vi "ControlShooter.vi"(1 "State":T2) -> (0 "To Shooter\nSolenoid Loop":T1=enum."Forward")   [LabVIEW 2013]
uses:
  typedefs/subStates.ctl
  <vilib>/Rock Robotics/WPI/Solenoid/WPI_SolenoidGetEnum.vi
  <vilib>/Rock Robotics/WPI/Solenoid/WPI_SolenoidValue.ctl
  typedefs/fg_typedef.ctl
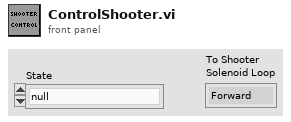
[diagram p1: front panel]
types:
  T1 = typedef "WPI_SolenoidValue.ctl" = enum16{"Off", "On", "Forward", "Reverse"}
  T2 = typedef "subStates.ctl" = enum16{"null", "wait", "driver control", "auto", "manual override", "hold position", "rotate", "pickup", "pass", "load", "goto shoot", "shoot high goal", "shoot low goal", "cancel arm", "cancel shooter", "end"}
  T3 = typedef "fg_typedef.ctl" = enum16{"Get", "Set"}
  T4 = typedef "WPI_DigitalInputDevRef.ctl" = cluster{"DevStatus":errorcluster, "DIO Channel":T5, "Digital Module":T6}
  T5 = typedef "FPGA_DIOChannel.ctl" = enum8{"DIO 1", "DIO 2", "DIO 3", "DIO 4", "DIO 5", "DIO 6", "DIO 7", "DIO 8", "DIO 9", "DIO 10", "DIO 11", "DIO 12", "DIO 13", "DIO 14", "Invalid"}
  T6 = typedef "FPGA_TypedefDigitalModule.ctl" = enum16{"Digital Module 1", "Digital Module 2"}
  T7 = typedef "WPI_SolenoidDevRef.ctl" = cluster{"DevStatus":errorcluster, "Solenoid Module":T8, "Forward Solenoid Channel":T9, "Reverse Solenoid Channel":T9}
  T8 = typedef "FPGA_TypedefSolenoidModule.ctl" = enum16{"Solenoid Module 1", "Solenoid Module 2"}
  T9 = typedef "WPI_SolenoidChannel.ctl" = enum8{"Solenoid 1", "Solenoid 2", "Solenoid 3", "Solenoid 4", "Solenoid 5", "Solenoid 6", "Solenoid 7", "Solenoid 8", "Invalid"}
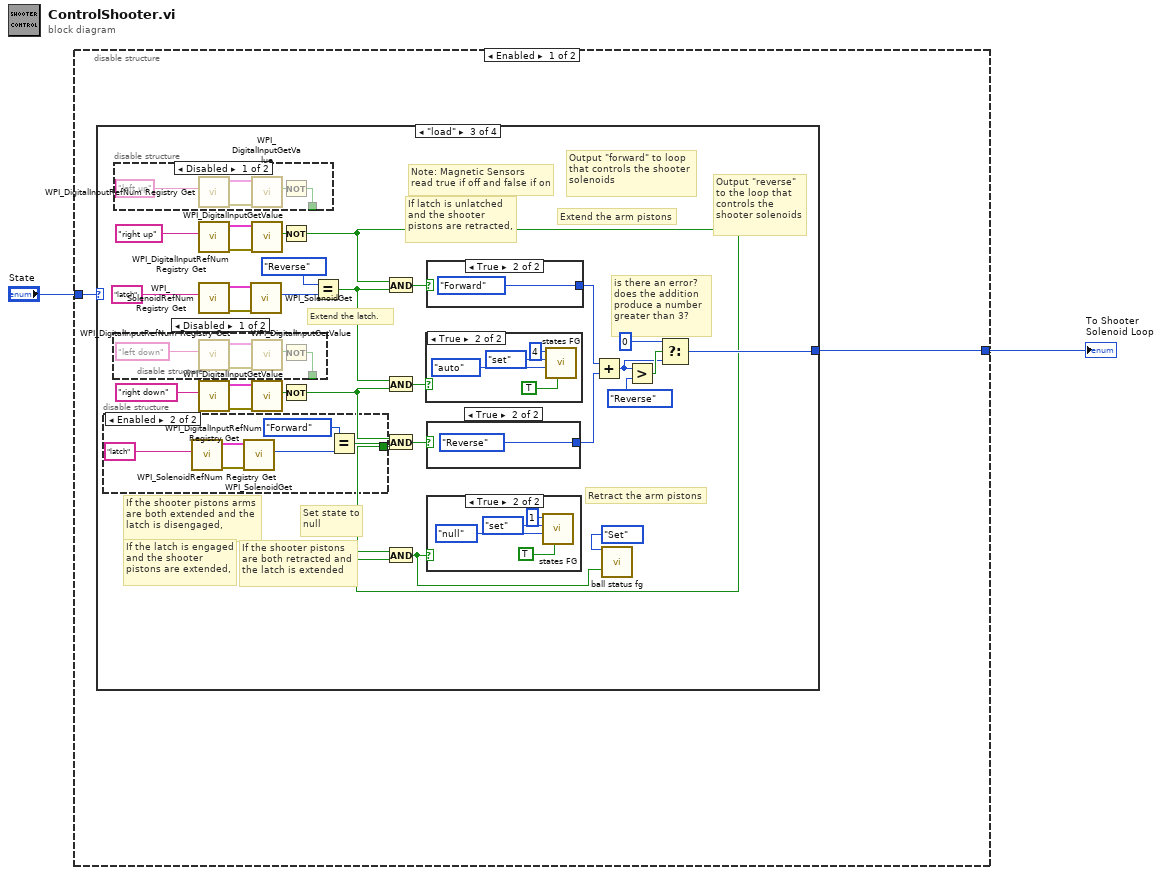
[diagram p0: block diagram]
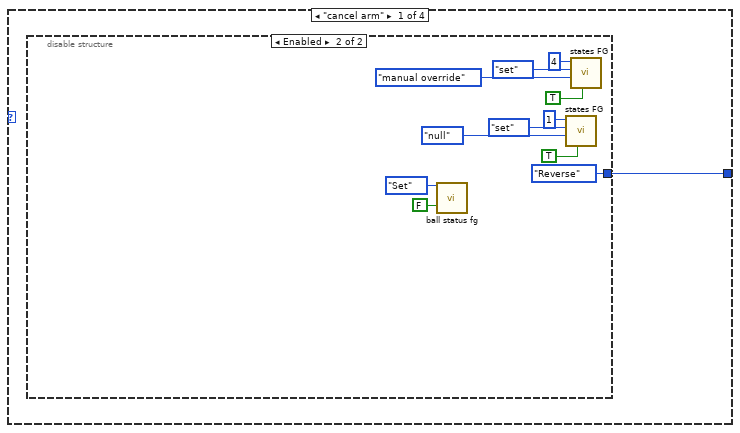
[diagram p2: hidden frame]
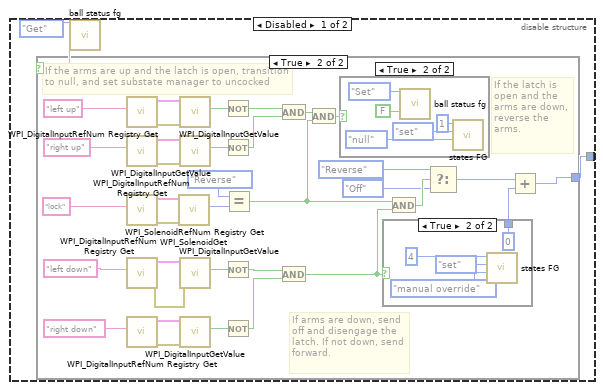
[diagram p3: hidden frame]
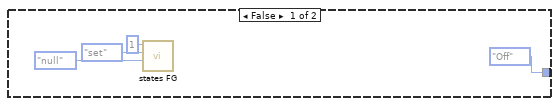
[diagram p4: hidden frame]
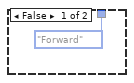
[diagram p6: hidden frame]
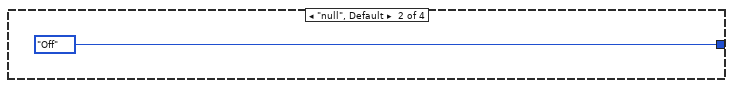
[diagram p7: hidden frame]
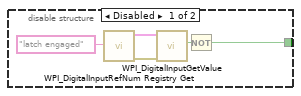
[diagram p8: hidden frame]
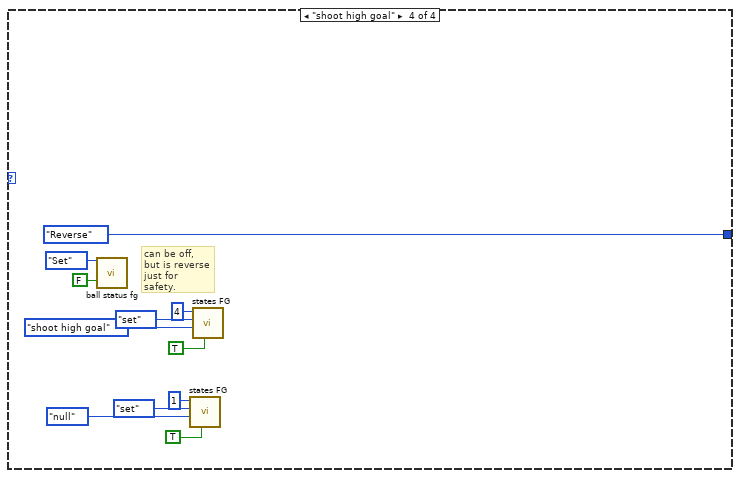
[diagram p15: hidden frame]
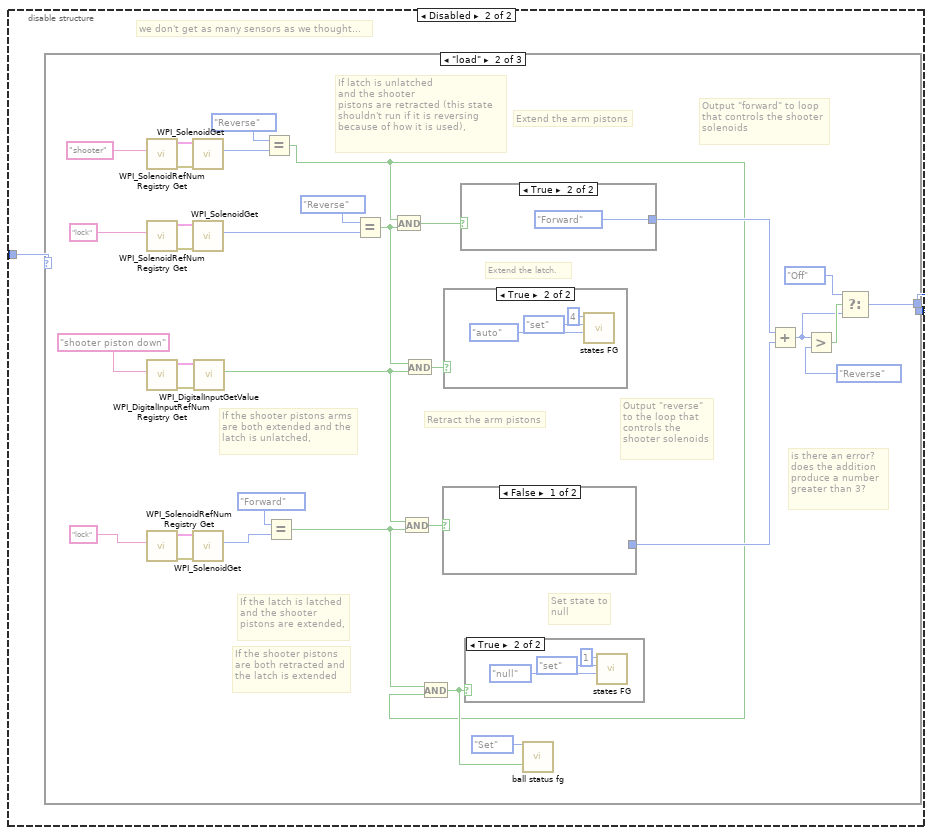
[diagram p16: hidden frame]
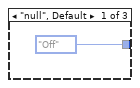
[diagram p17: hidden frame]
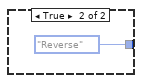
[diagram p19: hidden frame]
diagram:
  n1 = disable-structure shown="Enabled" {
    disable-tunnel: "State" -> [w4 w142]
    disable-tunnel: [w3 w141] -> w1
    frame Enabled {
      n2 = case shown="\"load\"" w4 {
        tunnel: [w5 WPI_SolenoidValue."Off" ("To Shooter\nSolenoid Loop") w78 WPI_SolenoidValue."Reverse" ("To Shooter\nSolenoid Loop")] -> w3
        frame "cancel arm" {
          n3 = disable-structure shown="Enabled" {
            disable-tunnel: [w6 WPI_SolenoidValue."Reverse" ("To Shooter\nSolenoid Loop")] -> w5
            frame Disabled {
              n4 = call "ball status fg.vi"("Menu"=fg_typedef."Get") -> (18:w7)  [unwired: 17 in, 1 out]
              n5 = case shown="True" w7 {
                tunnel: [WPI_SolenoidValue."Off" ("To Shooter\nSolenoid Loop") w16] -> w6
                frame False {
                  n6 = call "states FG.vi"("subState in"=subStates."null", "menu (get)"=enum16{"set", "get"}."set", "Loop ID"=1) -> ()  [unwired: 5 in, 4 out]
                }
                frame True {
                  # "If the arms are up and the latch is open, transition\nto null, and set substate manager to uncocked"
                  # "If the latch is\nopen and the\narms are down,\nreverse the\narms."
                  # "If arms are down, send\noff and disengage the\nlatch. If not down, send\nforward."
                  n7 = call <vilib>:"WPI_DigitalInputRefNum Registry Get.vi"("refnum name"="left up") -> ("error out"=w34:errorcluster, "DigitalInputDevRef"=w33:T4)  [unwired: 9 in]
                  n8 = call <vilib>:"WPI_DigitalInputRefNum Registry Get.vi"("refnum name"="right up") -> ("error out"=w31:errorcluster, "DigitalInputDevRef"=w30:T4)  [unwired: 9 in]
                  n9 = call <vilib>:"WPI_SolenoidRefNum Registry Get.vi"("refnum name"="lock") -> ("error out"=w27:errorcluster, "SolenoidDevRef"=w28:T7)  [unwired: 9 in]
                  n10 = call <vilib>:"WPI_DigitalInputRefNum Registry Get.vi"("refnum name"="left down") -> ("error out"=w37:errorcluster, "DigitalInputDevRef"=w36:T4)  [unwired: 9 in]
                  n11 = call <vilib>:"WPI_DigitalInputRefNum Registry Get.vi"("refnum name"="right down") -> ("error out"=w40:errorcluster, "DigitalInputDevRef"=w39:T4)  [unwired: 9 in]
                  n12 = call-poly <vilib>:"WPI_SolenoidGet.vi"("error in (no error)"=w27, "SolenoidDevRef"=w28) -> ("Value"=w46:T1)  [unwired: 7 in, 2 out]
                  n13 = call <vilib>:"WPI_DigitalInputGetValue.vi"("error in (no error)"=w34, "DigitalInputDevRef"=w33) -> ("Value"=w45:bool)  [unwired: 7 in, 2 out]
                  n14 = call <vilib>:"WPI_DigitalInputGetValue.vi"("error in (no error)"=w31, "DigitalInputDevRef"=w30) -> ("Value"=w44:bool)  [unwired: 7 in, 2 out]
                  n15 = call <vilib>:"WPI_DigitalInputGetValue.vi"("error in (no error)"=w37, "DigitalInputDevRef"=w36) -> ("Value"=w43:bool)  [unwired: 7 in, 2 out]
                  n16 = call <vilib>:"WPI_DigitalInputGetValue.vi"("error in (no error)"=w40, "DigitalInputDevRef"=w39) -> ("Value"=w42:bool)  [unwired: 7 in, 2 out]
                  n17 = Not(x=w45) -> (.not. x?=w25:bool)
                  n18 = Not(x=w44) -> (.not. x?=w26:bool)
                  n19 = Not(x=w43) -> (.not. x?=w23:bool)
                  n20 = Not(x=w42) -> (.not. x?=w24:bool)
                  n21 = Equal?(x=WPI_SolenoidValue."Reverse", y=w46) -> (x = y?=w14:bool)
                  n22 = And(x=w25, y=w26) -> (x .and. y?=w15:bool)
                  n23 = And(x=w23, y=w24) -> (x .and. y?=w22:bool)
                  n24 = And(x=w15, y=w14) -> (x .and. y?=w13:bool)
                  n25 = case shown="True" w13 {
                    frame False {
                    }
                    frame True {
                      n26 = call "ball status fg.vi"("Menu"=fg_typedef."Set", 4:FALSE ("Shooter Cocked")) -> ()  [unwired: 17 in, 1 out]
                      n27 = call "states FG.vi"("subState in"=subStates."null", "menu (get)"=enum16{"set", "get"}."set", "Loop ID"=1) -> ()  [unwired: 5 in, 4 out]
                    }
                  }
                  n28 = case shown="True" w22 {
                    tunnel: [WPI_SolenoidValue."Forward" ("To Shooter\nSolenoid Loop") 0] -> w21
                    frame False {
                    }
                    frame True {
                      n29 = call "states FG.vi"("subState in"=subStates."manual override", "menu (get)"=enum16{"set", "get"}."set", "Loop ID"=4) -> ()  [unwired: 5 in, 4 out]
                    }
                  }
                  n30 = And(x=w14, y=w22) -> (x .and. y?=w20:bool)
                  n31 = Select(t=WPI_SolenoidValue."Reverse" ("To Shooter\nSolenoid Loop"), s=w20, f=WPI_SolenoidValue."Off") -> (s? t:f=w18:T1)
                  n32 = Add(x=w18, y=w21) -> (x+y=w16:i32)
                }
              }
            }
            frame Enabled {
              n33 = call "ball status fg.vi"("Menu"=fg_typedef."Set", 4:FALSE ("Shooter Cocked")) -> ()  [unwired: 17 in, 1 out]
              n34 = call "states FG.vi"("exit in"=TRUE, "subState in"=subStates."null", "menu (get)"=enum16{"set", "get"}."set", "Loop ID"=1) -> ()  [unwired: 4 in, 4 out]
              n35 = call "states FG.vi"("exit in"=TRUE, "subState in"=subStates."manual override", "menu (get)"=enum16{"set", "get"}."set", "Loop ID"=4) -> ()  [unwired: 4 in, 4 out]
            }
          }
        }
        frame "null", Default {
        }
        frame "load" {
          # "Note: Magnetic Sensors\nread true if off and false if on"
          # "is there an error?\ndoes the addition\nproduce a number \ngreater than 3?"
          # "Output \"reverse\"\nto the loop that\ncontrols the\nshooter solenoids"
          # "Output \"forward\" to loop\nthat controls the shooter\nsolenoids"
          # "Set state to\nnull"
          # "If the shooter pistons\nare both retracted and\nthe latch is extended"
          # "If the latch is engaged\nand the shooter\npistons are extended,"
          # "Retract the arm pistons"
          # "If latch is unlatched\nand the shooter\npistons are retracted,"
          # "Extend the latch."
          # "If the shooter pistons arms\nare both extended and the\nlatch is disengaged,"
          # "Extend the arm pistons"
          n36 = disable-structure shown="Enabled" {
            disable-tunnel: [w99 w106] -> w74
            frame Disabled {
              n37 = call <vilib>:"WPI_DigitalInputRefNum Registry Get.vi"("refnum name"="latch engaged") -> ("error out"=w101:errorcluster, "DigitalInputDevRef"=w102:T4)  [unwired: 9 in]
              n38 = call <vilib>:"WPI_DigitalInputGetValue.vi"("error in (no error)"=w101, "DigitalInputDevRef"=w102) -> ("Value"=w100:bool)  [unwired: 7 in, 2 out]
              n39 = Not(x=w100) -> (.not. x?=w99:bool)
            }
            frame Enabled {
              n40 = call <vilib>:"WPI_SolenoidRefNum Registry Get.vi"("refnum name"="latch") -> ("error out"=w107:errorcluster, "SolenoidDevRef"=w108:T7)  [unwired: 9 in]
              n41 = call-poly <vilib>:"WPI_SolenoidGet.vi"("error in (no error)"=w107, "SolenoidDevRef"=w108) -> ("Value"=w105:T1)  [unwired: 7 in, 2 out]
              n42 = Equal?(x=WPI_SolenoidValue."Forward", y=w105) -> (x = y?=w106:bool)
            }
          }
          n43 = disable-structure shown="Disabled" {
            disable-tunnel: [w110 _] -> _
            frame Disabled {
              n44 = call <vilib>:"WPI_DigitalInputRefNum Registry Get.vi"("refnum name"="left down") -> ("error out"=w113:errorcluster, "DigitalInputDevRef"=w114:T4)  [unwired: 9 in]
              n45 = call <vilib>:"WPI_DigitalInputGetValue.vi"("error in (no error)"=w113, "DigitalInputDevRef"=w114) -> ("Value"=w111:bool)  [unwired: 7 in, 2 out]
              n46 = Not(x=w111) -> (.not. x?=w110:bool)
            }
            frame Enabled {
            }
          }
          n47 = disable-structure shown="Disabled" {
            disable-tunnel: [w115 _] -> _
            frame Disabled {
              n48 = call <vilib>:"WPI_DigitalInputRefNum Registry Get.vi"("refnum name"="left up") -> ("error out"=w118:errorcluster, "DigitalInputDevRef"=w119:T4)  [unwired: 9 in]
              n49 = call <vilib>:"WPI_DigitalInputGetValue.vi"("error in (no error)"=w118, "DigitalInputDevRef"=w119) -> ("Value"=w116:bool)  [unwired: 7 in, 2 out]
              n50 = Not(x=w116) -> (.not. x?=w115:bool)
            }
            frame Enabled {
            }
          }
          n51 = call <vilib>:"WPI_DigitalInputRefNum Registry Get.vi"("refnum name"="right up") -> ("error out"=w92:errorcluster, "DigitalInputDevRef"=w93:T4)  [unwired: 9 in]
          n52 = call <vilib>:"WPI_SolenoidRefNum Registry Get.vi"("refnum name"="latch") -> ("error out"=w98:errorcluster, "SolenoidDevRef"=w97:T7)  [unwired: 9 in]
          n53 = call <vilib>:"WPI_DigitalInputRefNum Registry Get.vi"("refnum name"="right down") -> ("error out"=w87:errorcluster, "DigitalInputDevRef"=w88:T4)  [unwired: 9 in]
          n54 = call-poly <vilib>:"WPI_SolenoidGet.vi"("error in (no error)"=w98, "SolenoidDevRef"=w97) -> ("Value"=w95:T1)  [unwired: 7 in, 2 out]
          n55 = call <vilib>:"WPI_DigitalInputGetValue.vi"("error in (no error)"=w92, "DigitalInputDevRef"=w93) -> ("Value"=w72:bool)  [unwired: 7 in, 2 out]
          n56 = call <vilib>:"WPI_DigitalInputGetValue.vi"("error in (no error)"=w87, "DigitalInputDevRef"=w88) -> ("Value"=w73:bool)  [unwired: 7 in, 2 out]
          n57 = Not(x=w72) -> (.not. x?=w71:bool)
          n58 = Not(x=w73) -> (.not. x?=w70:bool)
          n59 = Equal?(x=WPI_SolenoidValue."Reverse", y=w95) -> (x = y?=w84:bool)
          n60 = And(x=w71, y=w84) -> (x .and. y?=w90:bool)
          n61 = And(x=w84, y=w70) -> (x .and. y?=w89:bool)
          n62 = And(x=w70, y=w74) -> (x .and. y?=w85:bool)
          n63 = And(x=w74, y=w71) -> (x .and. y?=w75:bool)
          n64 = case shown="True" w89 {
            frame False {
            }
            frame True {
              n65 = call "states FG.vi"("exit in"=TRUE, "subState in"=subStates."auto", "menu (get)"=enum16{"set", "get"}."set", "Loop ID"=4) -> ()  [unwired: 4 in, 4 out]
            }
          }
          n66 = case shown="True" w90 {
            tunnel: [_ WPI_SolenoidValue."Forward" ("Value")] -> w83
            frame False {
            }
            frame True {
            }
          }
          n67 = case shown="True" w85 {
            tunnel: [_ WPI_SolenoidValue."Reverse" ("Value")] -> w77
            frame False {
            }
            frame True {
            }
          }
          n68 = case shown="True" w75 {
            frame False {
            }
            frame True {
              n69 = call "states FG.vi"("exit in"=TRUE, "subState in"=subStates."null", "menu (get)"=enum16{"set", "get"}."set", "Loop ID"=1) -> ()  [unwired: 4 in, 4 out]
            }
          }
          n70 = Add(x=w83, y=w77) -> (x+y=w80:u16)
          n71 = call "ball status fg.vi"("Menu"=fg_typedef."Set", 4:w75) -> ()  [unwired: 17 in, 1 out]
          n72 = Greater?(x=w80, y=WPI_SolenoidValue."Reverse" ("Value")) -> (0:w81:bool)
          n73 = Select(t=0, s=w81, f=w80) -> (s? t:f=w78:i32)
        }
        frame "shoot high goal" {
          # "can be off,\nbut is reverse\njust for safety."
          n74 = call "ball status fg.vi"("Menu"=fg_typedef."Set", 4:FALSE ("Shooter Cocked")) -> ()  [unwired: 17 in, 1 out]
          n75 = call "states FG.vi"("exit in"=TRUE, "subState in"=subStates."null", "menu (get)"=enum16{"set", "get"}."set", "Loop ID"=1) -> ()  [unwired: 4 in, 4 out]
          n76 = call "states FG.vi"("exit in"=TRUE, "subState in"=subStates."shoot high goal", "menu (get)"=enum16{"set", "get"}."set", "Loop ID"=4) -> ()  [unwired: 4 in, 4 out]
        }
      }
    }
    frame Disabled {
      # "we don't get as many sensors as we thought..."
      n77 = case shown="\"load\"" w142 {
        tunnel: [WPI_SolenoidValue."Off" ("To Shooter\nSolenoid Loop") w155 WPI_SolenoidValue."Off" ("To Shooter\nSolenoid Loop")] -> w141
        frame "null", Default {
        }
        frame "load" {
          # "is there an error?\ndoes the addition\nproduce a number \ngreater than 3?"
          # "Output \"reverse\"\nto the loop that\ncontrols the\nshooter solenoids"
          # "Output \"forward\" to loop\nthat controls the shooter\nsolenoids"
          # "Set state to\nnull"
          # "If the shooter pistons\nare both retracted and\nthe latch is extended"
          # "If the latch is latched\nand the shooter\npistons are extended,"
          # "Retract the arm pistons"
          # "If latch is unlatched\nand the shooter\npistons are retracted (this state shouldn't run if it is reversing because of how it is used),"
          # "Extend the latch."
          # "If the shooter pistons arms\nare both extended and the\nlatch is unlatched,"
          # "Extend the arm pistons"
          n78 = call <vilib>:"WPI_SolenoidRefNum Registry Get.vi"("refnum name"="shooter") -> ("error out"=w147:errorcluster, "SolenoidDevRef"=w148:T7)  [unwired: 9 in]
          n79 = call <vilib>:"WPI_SolenoidRefNum Registry Get.vi"("refnum name"="lock") -> ("error out"=w177:errorcluster, "SolenoidDevRef"=w176:T7)  [unwired: 9 in]
          n80 = call <vilib>:"WPI_DigitalInputRefNum Registry Get.vi"("refnum name"="shooter piston down") -> ("error out"=w169:errorcluster, "DigitalInputDevRef"=w170:T4)  [unwired: 9 in]
          n81 = call <vilib>:"WPI_SolenoidRefNum Registry Get.vi"("refnum name"="lock") -> ("error out"=w167:errorcluster, "SolenoidDevRef"=w166:T7)  [unwired: 9 in]
          n82 = call-poly <vilib>:"WPI_SolenoidGet.vi"("error in (no error)"=w147, "SolenoidDevRef"=w148) -> ("Value"=w149:T1)  [unwired: 7 in, 2 out]
          n83 = call-poly <vilib>:"WPI_SolenoidGet.vi"("error in (no error)"=w177, "SolenoidDevRef"=w176) -> ("Value"=w174:T1)  [unwired: 7 in, 2 out]
          n84 = call-poly <vilib>:"WPI_SolenoidGet.vi"("error in (no error)"=w167, "SolenoidDevRef"=w166) -> ("Value"=w164:T1)  [unwired: 7 in, 2 out]
          n85 = call <vilib>:"WPI_DigitalInputGetValue.vi"("error in (no error)"=w169, "DigitalInputDevRef"=w170) -> ("Value"=w151:bool)  [unwired: 7 in, 2 out]
          n86 = Equal?(x=WPI_SolenoidValue."Reverse", y=w149) -> (x = y?=w145:bool)
          n87 = Equal?(x=WPI_SolenoidValue."Forward", y=w164) -> (x = y?=w160:bool)
          n88 = Equal?(x=WPI_SolenoidValue."Reverse", y=w174) -> (x = y?=w161:bool)
          n89 = And(x=w145, y=w161) -> (x .and. y?=w172:bool)
          n90 = And(x=w151, y=w160) -> (x .and. y?=w162:bool)
          n91 = And(x=w161, y=w151) -> (x .and. y?=w171:bool)
          n92 = And(x=w160, y=w145) -> (x .and. y?=w152:bool)
          n93 = case shown="False" w162 {
            tunnel: [_ WPI_SolenoidValue."Reverse" ("Value")] -> w154
            frame False {
            }
            frame True {
            }
          }
          n94 = case shown="True" w171 {
            frame False {
            }
            frame True {
              n95 = call "states FG.vi"("subState in"=subStates."auto", "menu (get)"=enum16{"set", "get"}."set", "Loop ID"=4) -> ()  [unwired: 5 in, 4 out]
            }
          }
          n96 = case shown="True" w172 {
            tunnel: [_ WPI_SolenoidValue."Forward" ("Value")] -> w159
            frame False {
            }
            frame True {
            }
          }
          n97 = case shown="True" w152 {
            frame False {
            }
            frame True {
              n98 = call "states FG.vi"("subState in"=subStates."null", "menu (get)"=enum16{"set", "get"}."set", "Loop ID"=1) -> ()  [unwired: 5 in, 4 out]
            }
          }
          n99 = call "ball status fg.vi"("Menu"=fg_typedef."Set", 4:w152) -> ()  [unwired: 17 in, 1 out]
          n100 = Add(x=w159, y=w154) -> (x+y=w156:u16)
          n101 = Greater?(x=w156, y=WPI_SolenoidValue."Reverse" ("Value")) -> (0:w157:bool)
          n102 = Select(t=WPI_SolenoidValue."Off" ("Value"), s=w157, f=w156) -> (s? t:f=w155:u16)
        }
        frame "shoot high goal" {
          n103 = call "states FG.vi"("subState in"=subStates."null", "menu (get)"=enum16{"set", "get"}."set", "Loop ID"=1) -> ()  [unwired: 5 in, 4 out]
          n104 = call "states FG.vi"("subState in"=subStates."shoot high goal", "menu (get)"=enum16{"set", "get"}."set", "Loop ID"=4) -> ()  [unwired: 5 in, 4 out]
        }
      }
    }
  }
  "To Shooter\nSolenoid Loop" <- w1
